vi "Set DDS Amplitude Mv.vi"(10 "amplitdude":i32, 11 "channel_index":u8) -> ()   [LabVIEW 2021, in "vmmso.lvlib"]
doc: "DLL_API void WINAPI SetDDSAmplitudeMv(unsigned char channel_index, int amplitdude);"
uses:
  vmmso.lvlib
  vmmso.dll
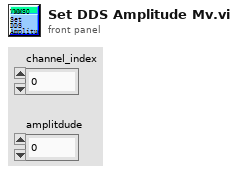
[diagram p1: front panel]
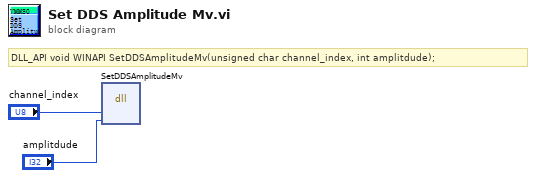
[diagram p0: block diagram]
diagram:
  # "DLL_API void WINAPI SetDDSAmplitudeMv(unsigned char channel_index, int amplitdude);"
  n1 = dll-call lib="D:/labviewdemo/LabviewDemo 21/vmmso/vmmso.*" fn="SetDDSAmplitudeMv"("channel_index"="channel_index", "amplitdude"="amplitdude") -> ()  [unwired: 6 in, 2 out]
